vi "Build Macro Step.vi"(11 "Prompt for Step FP Data":T5={"Step Type"=enum."Mouse Move", "Control Name"="", "Delay"=0, "Key"=65, "Repeat"=0, "RClick?"=FALSE, "App/Window Name"="", "X"=0, "Y"=0, "Notes"="", "Assertion Type"=enum."Control Position", "Assertion Parameters"=variant, "Disabled"=enum."Enabled", "Visible"=enum."Visible", "Left"=0, "Top"=0, "Width"=0, "Height"=0, "Expected Image"={"image type"=0, "image depth"=0, "image"=[], "mask"=[], "colors"=[], "Rectangle"={"left"=0, "top"=0, "right"=0, "bottom"=0}}}) -> (3 "Step":T1={"Type"=enum."Mouse Move", "X"=0, "Y"=0, "Delay"=0, "Key"=65, "Repeat"=0, "RClick?"=FALSE, "App/Window Name"="", "Notes"="", "Assertion Type"=enum."Control Position", "Control Name"="", "Disabled"=enum."Enabled", "Visible"=enum."Visible", "Left"=0, "Top"=0, "Width"=0, "Height"=0, "Expected Image"={"image type"=0, "image depth"=0, "image"=[], "mask"=[], "colors"=[], "Rectangle"={"left"=0, "top"=0, "right"=0, "bottom"=0}}})   [LabVIEW 2020, in "MacroAssert.lvlib"]
uses:
  MacroAssert.lvlib
  CTLs/Step Type V3.ctl
  CTLs/Assertion Type.ctl
  CTLs/Step V3.ctl
  <vilib>/picture/picture.llb/imagedata.ctl
  CTLs/Prompt for Step Front Panel Data.ctl
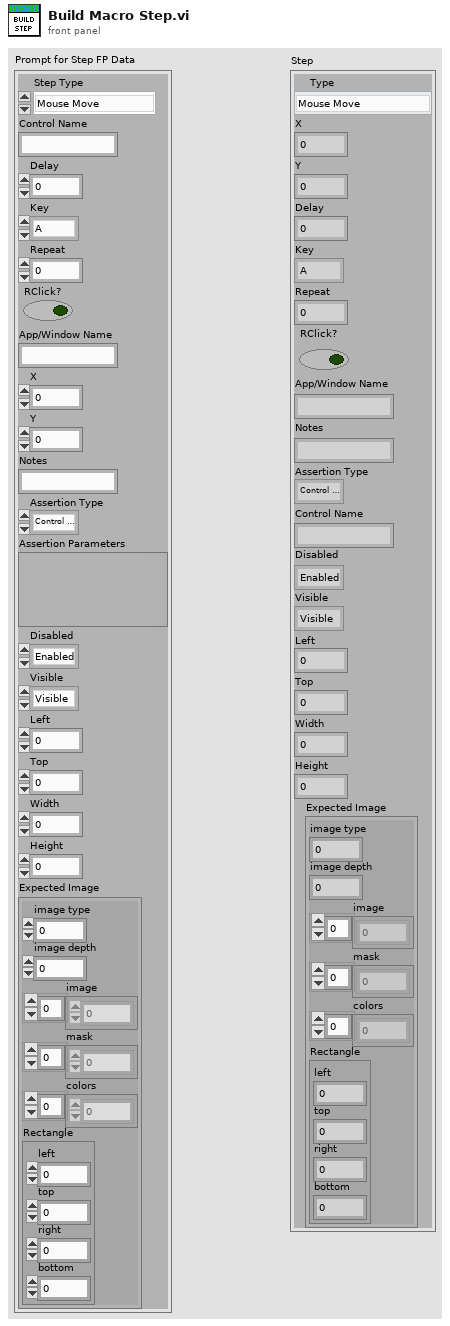
[diagram p1: front panel]
types:
  T1 = typedef "MacroAssert.lvlib/Step V3.ctl" = cluster{"Type":T2, "X":i32, "Y":i32, "Delay":i32, "Key":u8, "Repeat":i32, "RClick?":bool, "App/Window Name":string, "Notes":string, "Assertion Type":T3, "Control Name":string, "Disabled":enum8{"Enabled", "Disabled", "Disabled and Grayed Out"}, "Visible":enum16{"Visible", "Not Visible"}, "Left":i16, "Top":i16, "Width":i16, "Height":i16, "Expected Image":T4}
  T2 = typedef "MacroAssert.lvlib/Step Type V3.ctl" = enum16{"Mouse Move", "Mouse Click", "Key Press", "Wait", "Mouse Down", "Mouse Up", "Key Down", "Key Up", "Test Assertion", "Run Application", "Maximize Window", "Restore Window", "Minimize Window", "Close Window", "Bring Window to Front", "Send Window to Back"}
  T3 = typedef "MacroAssert.lvlib/Assertion Type.ctl" = enum16{"Control Position", "Control Visible", "Control Disabled", "Control Image"}
  T4 = typedef "imagedata.ctl" = cluster{"image type":i32, "image depth":i32, "image":u8[], "mask":u8[], "colors":u32[], "Rectangle":cluster{"left":i16, "top":i16, "right":i16, "bottom":i16}}
  T5 = typedef "MacroAssert.lvlib/Prompt for Step Front Panel Data.ctl" = cluster{"Step Type":T2, "Control Name":string, "Delay":i32, "Key":u8, "Repeat":i32, "RClick?":bool, "App/Window Name":string, "X":i32, "Y":i32, "Notes":string, "Assertion Type":T3, "Assertion Parameters":variant, "Disabled":enum8{"Enabled", "Disabled", "Disabled and Grayed Out"}, "Visible":enum16{"Visible", "Not Visible"}, "Left":i16, "Top":i16, "Width":i16, "Height":i16, "Expected Image":T4}
  T6 = enum8{"Enabled", "Disabled", "Disabled and Grayed Out"}
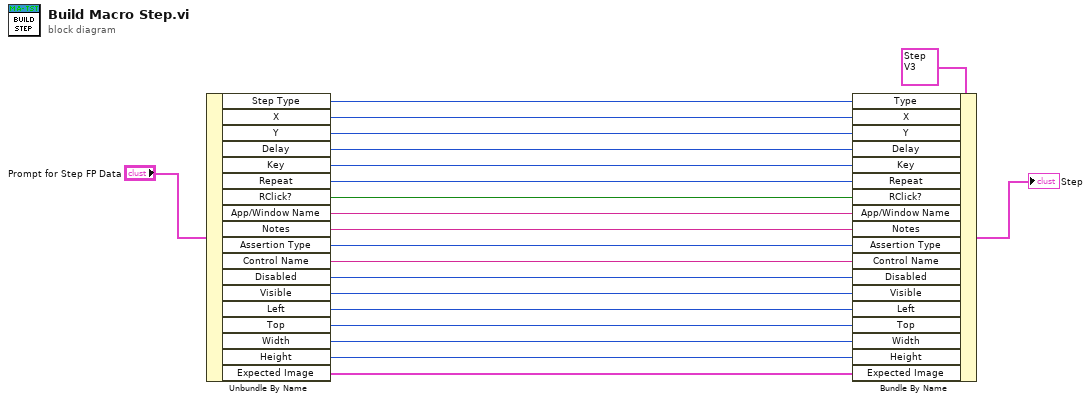
[diagram p0: block diagram]
diagram:
  n1 = Unbundle By Name("Prompt for Step FP Data") -> ("Step Type"=w20:T2, "X"=w19:i32, "Y"=w18:i32, "Delay"=w17:i32, "Key"=w16:u8, "Repeat"=w15:i32, "RClick?"=w14:bool, "App/Window Name"=w13:string, "Notes"=w12:string, "Assertion Type"=w11:T3, "Control Name"=w8:string, "Disabled"=w7:T6, "Visible"=w6:enum16{"Visible", "Not Visible"}, "Left"=w5:i16, "Top"=w4:i16, "Width"=w3:i16, "Height"=w2:i16, "Expected Image"=w1:T4)
  n2 = Bundle By Name(cluster=T1 {"Type"=enum."Mouse Move", "X"=0, "Y"=0, "Delay"=0, "Key"=65, "Repeat"=0, "RClick?"=FALSE, "App/Window Name"="", "Notes"="", "Assertion Type"=enum."Control Position", "Control Name"="", "Disabled"=enum."Enabled", "Visible"=enum."Visible", "Left"=0, "Top"=0, "Width"=0, "Height"=0, "Expected Image"={"image type"=0, "image depth"=0, "image"=[], "mask"=[], "colors"=[], "Rectangle"={"left"=0, "top"=0, "right"=0, "bottom"=0}}} ("Step"), "Type"=w20, "X"=w19, "Y"=w18, "Delay"=w17, "Key"=w16, "Repeat"=w15, "RClick?"=w14, "App/Window Name"=w13, "Notes"=w12, "Assertion Type"=w11, "Control Name"=w8, "Disabled"=w7, "Visible"=w6, "Left"=w5, "Top"=w4, "Width"=w3, "Height"=w2, "Expected Image"=w1) -> (→"Step":T1)
